vi "ArrayMaxMin.vi"(5 "符号取反？F":bool, 6 "in数组":sgl[](array[numeric])) -> (0 "MIN位置":i32, 1 "MIN":sgl, 2 "MAX位置":i32, 3 "MAX":sgl, 4 "平均值":sgl)   [LabVIEW 2018]
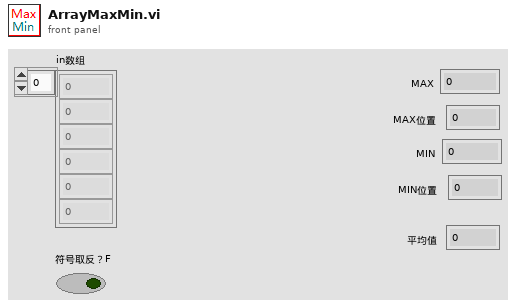
[diagram p1: front panel]
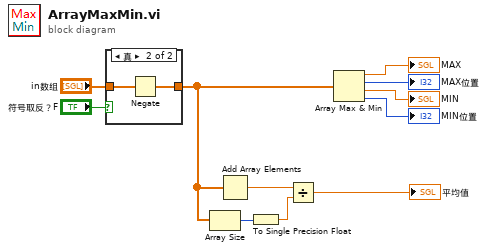
[diagram p0: block diagram]
diagram:
  n1 = case shown="真" "符号取反？F" {
    tunnel: [w12 w13] -> w4
    tunnel: "in数组" -> [w12 w14]
    frame False {
    }
    frame True {
      n2 = Negate(x=w14) -> (-x=w13:sgl[])
    }
  }
  n3 = Array Size(array=w4) -> (size(s)=w2:i32)
  n4 = Add Array Elements(numeric array=w4) -> (sum=w5:sgl)
  n5 = To Single Precision Float(number=w2) -> (single precision float=w3:sgl)
  n6 = Divide(x=w5, y=w3) -> (x/y=→"平均值":sgl)
  n7 = Array Max & Min(array=w4) -> (max value=→"MAX":sgl, max index (indices)=→"MAX位置":i32, min value=→"MIN":sgl, min index (indices)=→"MIN位置":i32)
